vi "Write exclusions.vi"(8 "error in":errorcluster, 10 "exclusions":string[](array[string]), 11 "VI modification in":refnum<class "VI modification.lvclass">) -> (0 "error out":errorcluster, 3 "VI modification out":refnum<class "VI modification.lvclass">)   [LabVIEW 2013, in "VI modification.lvclass"]
uses:
  VI modification.lvclass
  VI modification.lvclass/VI modification.ctl
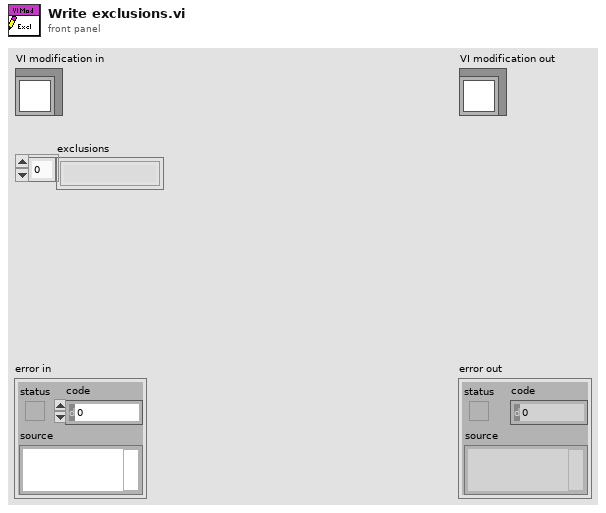
[diagram p1: front panel]
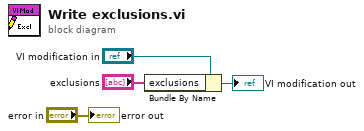
[diagram p0: block diagram]
diagram:
  n1 = Bundle By Name(cluster="VI modification in", "exclusions"="exclusions") -> (→"VI modification out":refnum<class "VI modification.lvclass">)
  "error out" <- "error in"
